vi "CAN Talon Position Control.vi"() -> ()   [LabVIEW 2015]
doc: "This example shows how to control motor speed using CAN Jaguar and a quadrature encoder. For details setting up and understanding CAN Jaguar, see the Can Jaguar Fundamentals tutorial accessable from the LabVIEW Getting Started Window.\n\nTo control the motor speed, a PID control loop runs on the Jaguar. Notice that the encoder is wired directly to the Jaguar. One advantage of this is that the PID control does not use resources on the roboRIO. One disadvantage is that the PID code cannot be viewed or changed. However, the control can be tuned by changing the PID Parameters.\n\nOn the diagram, notice that the PID tuning parameters are only applied once before the motor is enabled. To learn about changing PID parameters while the program is running, see the CAN Position Control Encoder example. Since the control loop runs on the Jaguar, the LabVIEW loop delay is set to a slow 100ms. In fact the only reason this loop needs to run is to send a new set speed and read the actual speed.\n\nCorrect tuning parameters for a PID controller are dependent on the complete system of the motor and the load. It will be difficult to tune this system if there is no load attached to the motor. While this example is not a PID tutorial, the following information may help in understanding how to tune your PID control system.\n\nP (proportional) depends on the present error, I (integral) on the accumulation of past errors, and D (derivative) is a prediction of future errors, based on the current rate of change. The proportional parameter (P) will reduce the rise time and will reduce, but never eliminate, the steady-state error. The integral parameter (I) will eliminate the steady-state error, but may make the transient response worse. The derivative parameter (D) will increase the stability of the system, reducing the overshoot, and improving the transient response. The effects of each parameter are summarized in a table on the front panel.\n\nThis example expects a USB cable connected from your development PC to the Type B USB Jack (next to the power input) on the roboRIO.\n\nThis example requires the Driver Station to be running with Teleoperated Enabled."
uses:
  <vilib>/Rock Robotics/WPI/CAN/TalonSRX/WPI_CANTalonSRX_APIControlMode.ctl
  <vilib>/Rock Robotics/WPI/CAN/TalonSRX/WPI_CANTalonSRX_APIFeedbackSelect.ctl
  <vilib>/Rock Robotics/WPI/Joystick/WPI_JoystickDeviceEnum.ctl
  <vilib>/Rock Robotics/WPI/MotorControl/WPI_MotorControlOpenCANTalonSRX.vi
panel:
  in  "Our Positioning":bool
  in  "stop 2":bool
  in  "F 2":dbl
  in  "I 2":dbl
  in  "D 2":dbl
  in  "P 2":dbl
  in  "Position Controller":dbl(knob) scale=0.0..1023.0
  in  "Reverse Feedback Sensor":bool
  in  "I":dbl
  in  "F":dbl=0.01
  in  "D":dbl=2.0
  in  "P":dbl=15.0
  in  "Master Device Number":u8
  in  "stop":bool
  # "Set these inputs before running."
  # "roboRIO Wiring Diagram"
  # "Tuning parameters"
  # "Slave Talon SRX"
  # "Master Talon SRX"
  # "Feed-Forward"
  # "Gnd"
  # "A"
  # "B"
  # "+5V"
  # "US Digital E4P Encoder"
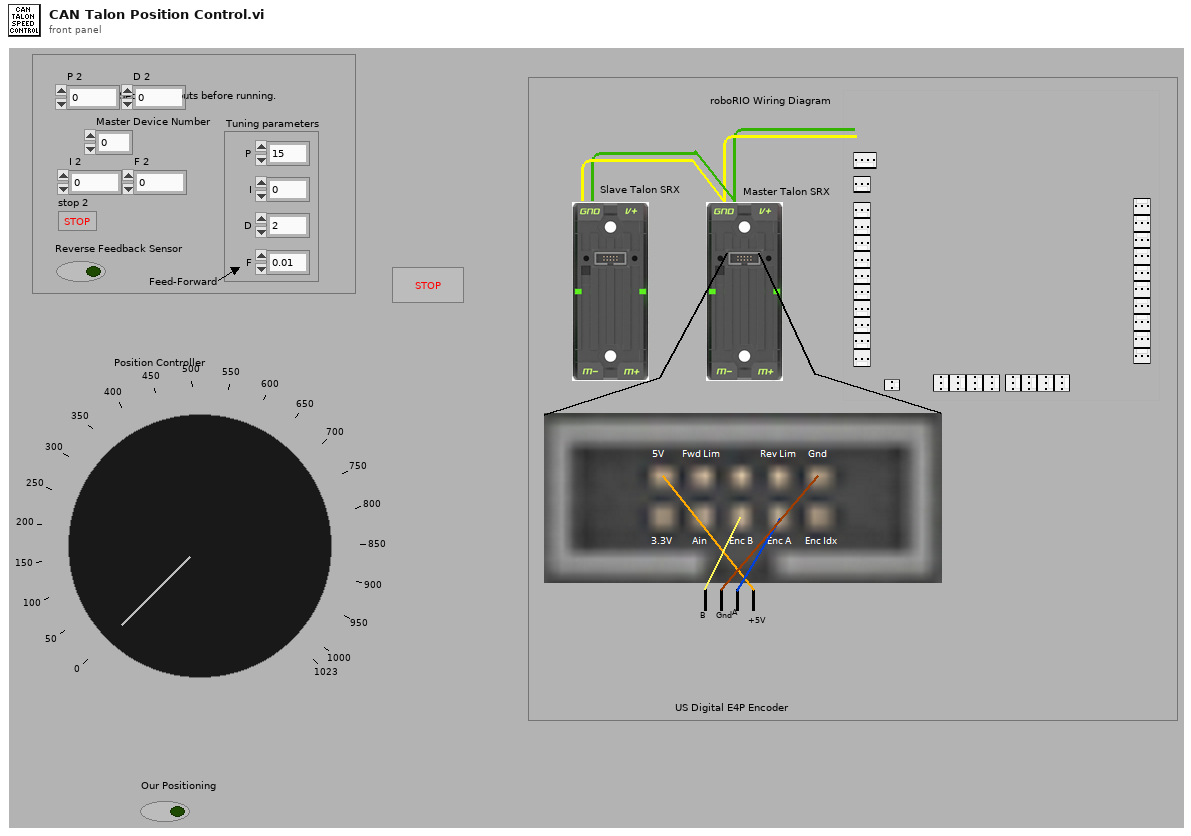
[diagram p1: front panel]
types:
  T1 = typedef "WPI_CANTalonSRX_APIFeedbackSelect.ctl" = enum16{"Digital Quadrature Encoder", "Analog Potentiometer", "Analog Encoder", "Count on Quad-A (Rising-Edge)", "Count on Quad-A (Falling-Edge)", "CTR Magnetic Enc (Absolute)", "CTR Magnetic Enc (Relative)", "Pulse Width"}
  T2 = typedef "WPI_CANTalonSRX_APIControlMode.ctl" = enum8{"Percent VBus", "Speed", "Position", "Slave", "Unchanged / Invalid", "Voltage Compensation", "Current", "Motion Profile"}
  T3 = typedef "WPI_JoystickDeviceEnum.ctl" = enum16{"USB 0", "USB 1", "USB 2", "USB 3", "USB 4", "USB 5"}
  T4 = typedef "WPI_MotorControlDeviceRef.ctl" = cluster{"DeviceStatus":errorcluster, "Type":T5, "PWM":cluster{"PWM Channel":T6, "DeadBand":T7}, "CAN":cluster{"Device Number":u8, "Control Mode":T8, "Semaphore":T9, "Max Vout":dbl, "TalonSRX Control Mode":T2}, "Invert":bool}
  T5 = typedef "WPI_MotorControlType.ctl" = enum16{"PWM", "CAN", "CANTalonSRX"}
  T6 = typedef "FPGA_DIOPWMChannel.ctl" = enum8{"PWM 0", "PWM 1", "PWM 2", "PWM 3", "PWM 4", "PWM 5", "PWM 6", "PWM 7", "PWM 8", "PWM 9", "PWM MXP 0", "PWM MXP 1", "PWM MXP 2", "PWM MXP 3", "PWM MXP 4", "PWM MXP 5", "PWM MXP 6", "PWM MXP 7", "PWM MXP 8", "PWM MXP 9", "Invalid"}
  T7 = typedef "WPI_PWMDeadband.ctl" = cluster{"Name":string, "maxPositivePwm":i32, "minPositivePwm":i32, "centerPwm":i32, "maxNegativePwm":i32, "minNegativePwm":i32, "angularRange":u16}
  T8 = typedef "WPI_CANJaguar_ControlMode.ctl" = enum8{"Percent VBus", "Current", "Speed", "Position", "Voltage"}
  T9 = typedef "Semaphore RefNum" = refnum<k1>
  T10 = typedef "WPI_JoystickDevRef.ctl" = cluster{"Device":T3}
  T11 = typedef "WPI_CANTalonSRX_GlobalStatus.ctl" = cluster{"Applied Throttle":dbl, "Module Enabled":bool, "CAN Error":errorcluster, "Closed Loop Error":dbl, "Forward Limit Switch Closed":bool, "Reverse Limit Switch Closed":bool, "Sensor Position":dbl, "Sensor Velocity":dbl, "Current":dbl, "Sticky Fault - Over Temp":bool, "Sticky Fault - Under Voltage":bool, "Sticky Fault - Forward Limit":bool, "Sticky Fault - Reverse Limit":bool, "Sticky Fault - Forward Soft Limit":bool, "Sticky Fault - Reverse Soft Limit":bool, "Brake is Enabled":bool, "Encoder Position":dbl, "Encoder Velocity":dbl, "Encoder Index Count":dbl, "Encoder A Pin State":bool, "Encoder B Pin State":bool, "Encoder Index Pin State":bool, "Analog In":dbl, "Analog In Velocity":dbl, "Temperature (C)":dbl, "Battery Voltage":dbl, "Control 5 Is Supported":bool, "Current Profile Slot Select":dbl, "Pos Div 8":bool, "Vel Div 4":bool, "Pulse Width Position":i32, "Pulse Width Velocity":i32, "Pulse Width Rise To Rise (us)":i32, "Pulse Width Rise To Fall (us)":i32, "Mot Prof Active Is Under Run":bool, "Mot Prof Active Has Under Run":bool, "Mot Prof Active Is Last":bool, "Mot Prof Active Velocity Only":bool, "Mot Prof Active Is Valid":bool, "Mot Prof Buffer Is Full":bool, "Mot Prof Active Profile Slot Select":i32, "Mot Prof NextID":i32, "Mot Prof Count":i32, "Mot Prof Active Velocity":dbl, "Mot Prof Active Position":dbl, "Mot Prof Output Enable":i32}
  T12 = cluster{"LeftX":dbl, "LeftY":dbl, "LTrigger":dbl, "RTrigger":dbl, "RightX":dbl, "RightY":dbl, "RightY 2":dbl, "RightX 2":dbl}
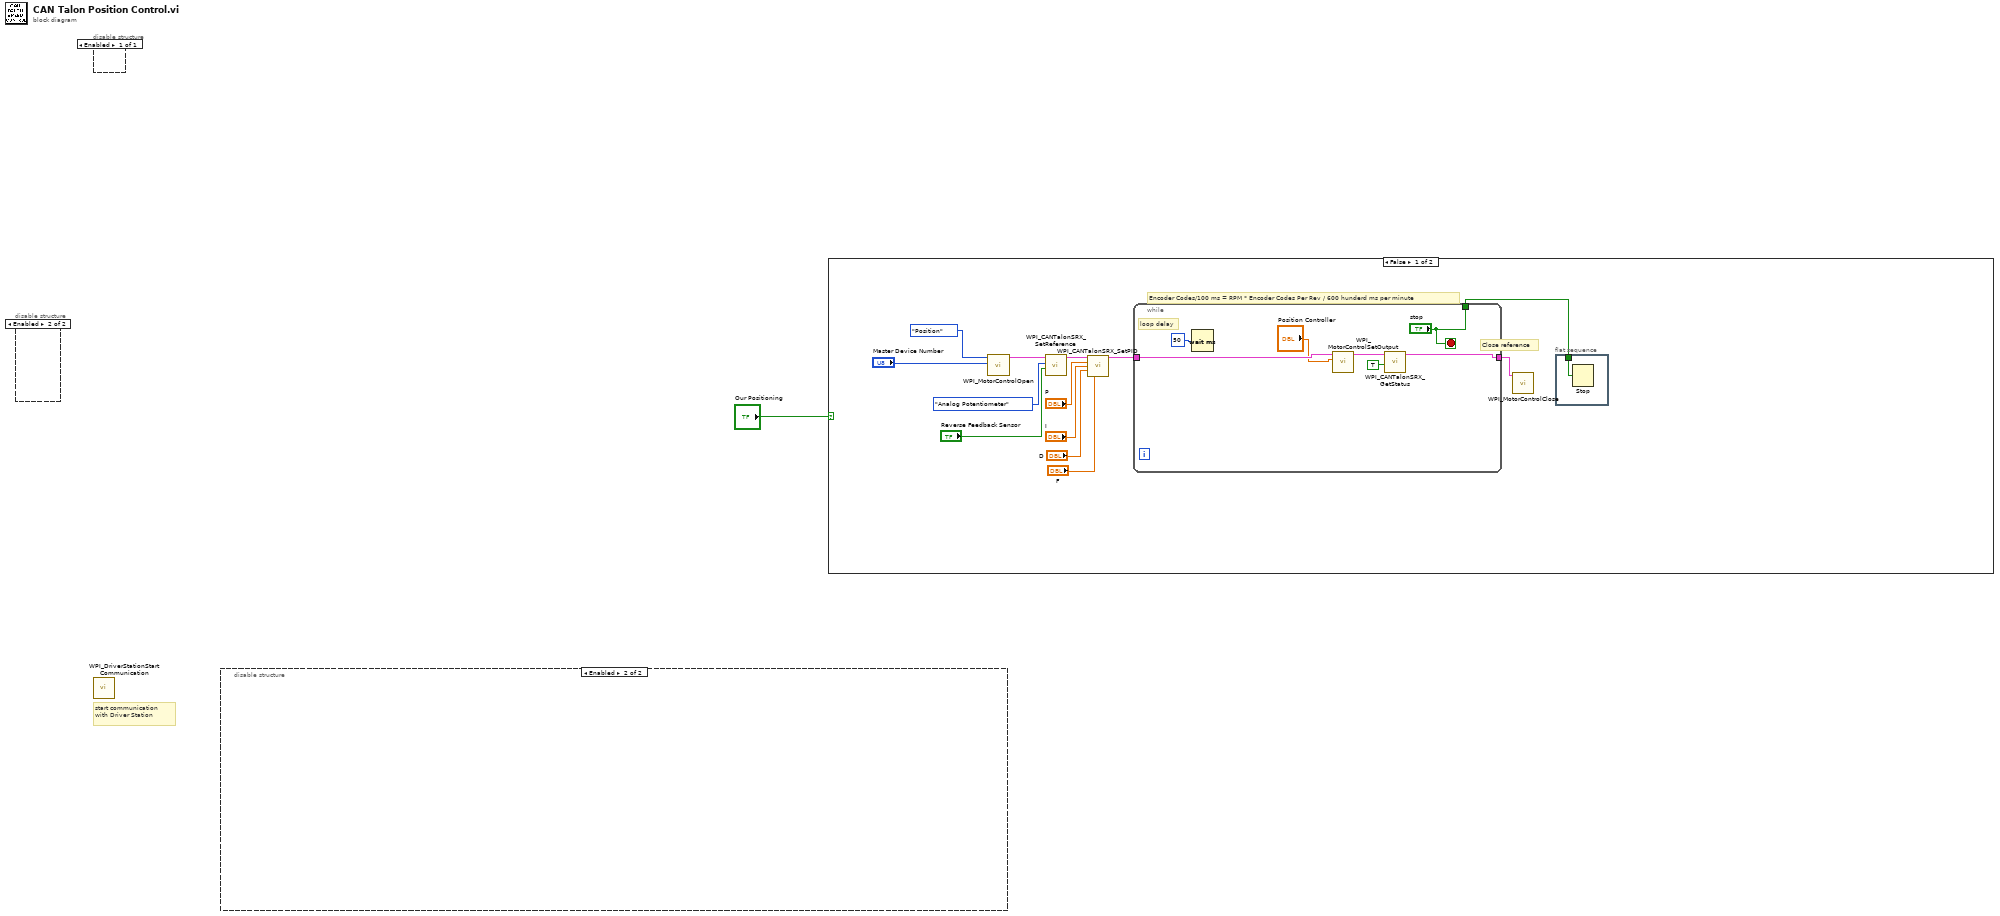
[diagram p0: block diagram]
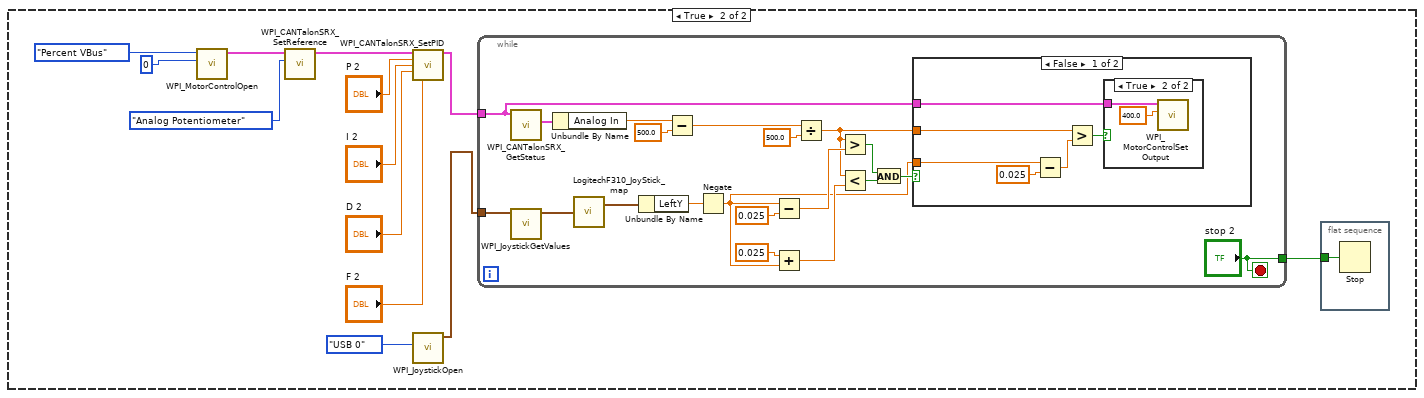
[diagram p2: hidden frame]
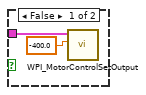
[diagram p3: hidden frame]
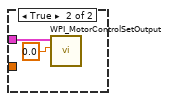
[diagram p4: hidden frame]
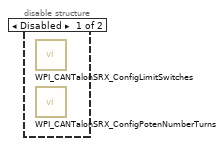
[diagram p6: hidden frame]
diagram:
  # "start communication with Driver Station"
  n1 = disable-structure shown="Enabled" {
    frame Disabled {
      n2 = call <vilib>:"WPI_CANTalonSRX_ConfigLimitSwitches.vi"() -> ()  [unwired: 14 in, 2 out]
      n3 = call <vilib>:"WPI_CANTalonSRX_ConfigPotenNumberTurns.vi"() -> ()  [unwired: 14 in, 2 out]
    }
    frame Enabled {
    }
  }
  n4 = disable-structure shown="Enabled" {
    frame Enabled {
    }
  }
  n5 = call <vilib>:"WPI_DriverStationStart Communication.vi"() -> ()  [unwired: 2 in, 10 out]
  n6 = disable-structure shown="Enabled" {
    frame Disabled {
    }
    frame Enabled {
    }
  }
  n7 = case shown="False" "Our Positioning" {
    frame False {
      # "Encoder Codes/100 ms = RPM * Encoder Codes Per Rev / 600 hunderd ms per minute"
      # "Close reference"
      n8 = call-poly <vilib>:"WPI_MotorControlOpen.vi"("Device Number"="Master Device Number", "Control Mode"=WPI_CANTalonSRX_APIControlMode."Position") -> ("MotorControlDeviceRef"=w11:T4)  [unwired: 3 in, 6 out]
      n9 = call <vilib>:"WPI_CANTalonSRX_SetReference.vi"("Reverse Feedback Sensor"="Reverse Feedback Sensor", "Feedback Reference"=WPI_CANTalonSRX_APIFeedbackSelect."Analog Potentiometer", "CAN Talon SRX Ref"=w11) -> ("CAN Talon SRX Ref"=w12:T4)  [unwired: 7 in, 1 out]
      n10 = call <vilib>:"WPI_CANTalonSRX_SetPID.vi"("CAN Talon SRX Ref"=w12, "P"="P", "I"="I", "D"="D", "F"="F") -> ("CAN Talon SRX Ref"=w4:T4)  [unwired: 9 in, 1 out]
      n11 = while {
        tunnel: ["stop"] -> w2
        tunnel: w4 -> [w20]
        tunnel: [w18] -> w3
        stop <- "stop" stop-if-true
        # "loop delay"
        n12 = Wait (ms)(milliseconds to wait=u32 50) -> ()  [unwired: 1 out]
        n13 = call <vilib>:"WPI_MotorControlSetOutput.vi"("Output"="Position Controller", "MotorControlDevRef"=w20) -> ("MotorControlDevRef"=w17:T4)  [unwired: 7 in, 2 out]
        n14 = call <vilib>:"WPI_CANTalonSRX_GetStatus.vi"("Clear Sticky Faults"=TRUE, "CAN Talon SRX Ref"=w17) -> ("CAN Talon SRX Ref"=w18:T4)  [unwired: 7 in, 2 out]
      }
      n15 = call <vilib>:"WPI_MotorControlClose.vi"("MotorControlDevRef"=w3) -> ()  [unwired: 10 in, 1 out]
      n16 = flat-sequence {
        tunnel: w2 -> [w15]
        frame #0 {
          n17 = Stop(stop? (T)=w15) -> ()
        }
      }
    }
    frame True {
      n18 = call-poly <vilib>:"WPI_MotorControlOpen.vi"("Device Number"=u8 0, "Control Mode"=WPI_CANTalonSRX_APIControlMode."Percent VBus") -> ("MotorControlDeviceRef"=w27:T4)  [unwired: 8 in, 1 out]
      n19 = call <vilib>:"WPI_CANTalonSRX_SetReference.vi"("Feedback Reference"=WPI_CANTalonSRX_APIFeedbackSelect."Analog Potentiometer", "CAN Talon SRX Ref"=w27) -> ("CAN Talon SRX Ref"=w29:T4)  [unwired: 8 in, 1 out]
      n20 = call <vilib>:"WPI_CANTalonSRX_SetPID.vi"("CAN Talon SRX Ref"=w29, "P"="P 2", "I"="I 2", "D"="D 2", "F"="F 2") -> ("CAN Talon SRX Ref"=w23:T4)  [unwired: 9 in, 1 out]
      n21 = call <vilib>:"WPI_JoystickOpen.vi"("JoystickDevice"=WPI_JoystickDeviceEnum."USB 0") -> ("JoystickDevRef"=w24:T10)  [unwired: 10 in]
      n22 = while {
        tunnel: w23 -> [w51]
        tunnel: w24 -> [w55]
        tunnel: ["stop 2"] -> w35
        stop <- "stop 2" stop-if-true
        n23 = call <vilib>:"WPI_CANTalonSRX_GetStatus.vi"("CAN Talon SRX Ref"=w51) -> ("Talon SRX Status"=w56:T11)  [unwired: 8 in, 2 out]
        n24 = call <vilib>:"WPI_JoystickGetValues.vi"("JoystickDevRef"=w55) -> ("JoystickDevRef"=w54:T10)  [unwired: 6 in, 4 out]
        n25 = Unbundle By Name(w56) -> ("Analog In"=w46:dbl)
        n26 = call "LogitechF310_JoyStick_map.vi"("JoystickDevRef"=w54) -> ("AxesCluster"=w53:T12)  [unwired: 1 out]
        n27 = Unbundle By Name(w53) -> ("LeftY"=w52:dbl)
        n28 = Subtract(x=w46, y=500.0) -> (x-y=w48:dbl)
        n29 = Negate(x=w52) -> (-x=w37:dbl)
        n30 = Subtract(x=w37, y=0.025) -> (x-y=w43:dbl)
        n31 = Add(x=0.025, y=w37) -> (x+y=w39:dbl)
        n32 = Divide(x=w48, y=500.0) -> (x/y=w40:dbl)
        n33 = Greater?(x=w40, y=w43) -> (0:w44:bool)
        n34 = Less?(x=w40, y=w39) -> (x < y?=w41:bool)
        n35 = And(x=w44, y=w41) -> (x .and. y?=w45:bool)
        n36 = case shown="False" w45 {
          tunnel: w40 -> [w62 _]
          tunnel: w37 -> [w61 _]
          tunnel: w51 -> [w59 w67]
          frame False {
            n37 = Subtract(x=w61, y=0.025) -> (x-y=w58:dbl)
            n38 = Greater?(x=w62, y=w58) -> (0:w60:bool)
            n39 = case shown="True" w60 {
              tunnel: w59 -> [w64 w66]
              frame False {
                n40 = call <vilib>:"WPI_MotorControlSetOutput.vi"("Output"=-400.0, "MotorControlDevRef"=w64) -> ()  [unwired: 7 in, 3 out]
              }
              frame True {
                n41 = call <vilib>:"WPI_MotorControlSetOutput.vi"("Output"=400.0, "MotorControlDevRef"=w66) -> ()  [unwired: 7 in, 3 out]
              }
            }
          }
          frame True {
            n42 = call <vilib>:"WPI_MotorControlSetOutput.vi"("Output"=0.0, "MotorControlDevRef"=w67) -> ()  [unwired: 7 in, 3 out]
          }
        }
      }
      n43 = flat-sequence {
        tunnel: w35 -> [w36]
        frame #0 {
          n44 = Stop(stop? (T)=w36) -> ()
        }
      }
    }
  }
